vi "Create Transfer Group.vi"(6 "Buffers":refnum<class "Buffers.lvclass">, 7 "id":i32, 8 "error in (no error)":errorcluster, 9 "direction":T2, 10 "cycle timing":T1, 11 "Transfers":refnum<class "Transfer.lvclass">[](array[class])) -> (0 "error out":errorcluster, 3 "Transfer Group out":refnum<class "Transfer Group.lvclass">)   [LabVIEW 2017, in "DSF Core.lvlib" / "Transfer Group.lvclass"]
uses:
  Transfer Group.lvclass
  Transfer/Transfer.lvclass
  DSF Configuration API/Public/Controls/DSF Direction.ctl
  DSF Configuration API/Public/Controls/DSF Timing Info.ctl
  Buffer/Buffers.lvclass
  Transfer Group.lvclass/Transfer Group.ctl
  Timing/Transfer Group Timing.lvclass
  DSF Core.lvlib
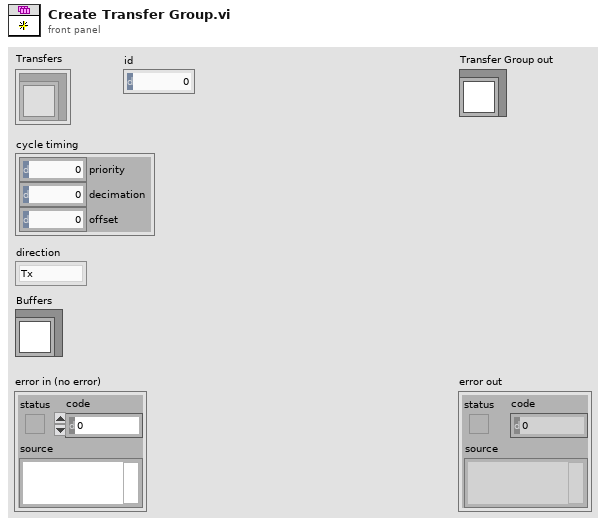
[diagram p1: front panel]
types:
  T1 = typedef "DSF Core.lvlib/DSF Timing Info.ctl" = cluster{"priority":u64, "decimation":u64, "offset":u64}
  T2 = typedef "DSF Core.lvlib/DSF Direction.ctl" = enum8{"Tx", "Rx"}
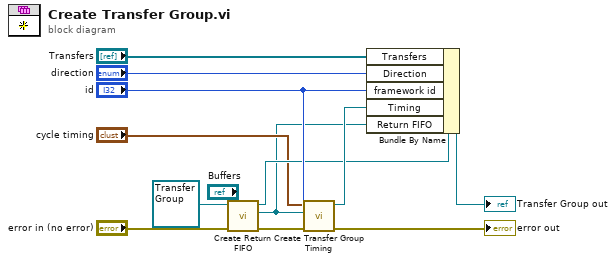
[diagram p0: block diagram]
diagram:
  n1 = call "Create Return FIFO.vi"("error in (no error)"="error in (no error)", "Transfer Group in"=refnum<class "Transfer Group.lvclass"> refnum ("Transfer Group type")) -> ("error out"=w6:errorcluster, "return fifo"=w1:refnum<k33>, "Transfer Group out"=w3:refnum<class "Transfer Group.lvclass">)  [unwired: 7 in]
  n2 = call "Create Transfer Group Timing.vi"("id"="id", "error in (no error)"=w6, "Return FIFO"=w1, "cycle timing"="cycle timing") -> ("error out"=→"error out":errorcluster, "Transfer Group Timing out"=w4:refnum<class "Transfer Group Timing.lvclass">)  [unwired: 6 in]
  n3 = Bundle By Name(cluster=w3, "Transfers"="Transfers", "Direction"="direction", "framework id"="id", "Timing"=w4, "Return FIFO"=w1) -> (→"Transfer Group out":refnum<class "Transfer Group.lvclass">)
